vi "ResizeGreyscale.vi"(7 "OpenCV Interpolation Flag":T1, 8 "error in (no error)":errorcluster, 9 "New Image Size":T2, 10 "Greyscale Destination Image":refnum<data-value>, 11 "Greyscale Source Image":refnum<data-value>) -> (0 "error out":errorcluster, 3 "Greyscale Destination Image (duplicate)":refnum<data-value>)   [LabVIEW 2020, in "g_ar_toolkit.image.lvlib"]
uses:
  g_ar_toolkit.image.lvlib
  g_ar_toolkit.common/Image Size (Integer).ctl
  Interpolation Mode.ctl
  eaa3f26c-b51e-4a69-9610-cf2aa5919b39.vi
  <vilib>/Utility/error.llb/Error Cluster From Error Code.vi
  g_ar_toolkit.common/g_ar_toolkit.common.lvlib
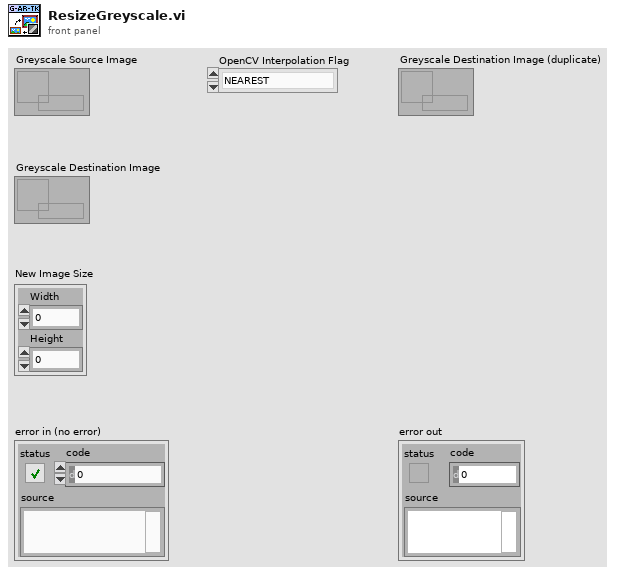
[diagram p1: front panel]
types:
  T1 = typedef "g_ar_toolkit.image.lvlib/Interpolation Mode.ctl" = enum8{"NEAREST", "LINEAR", "CUBIC", "AREA", "LANCZOS", "LINEAR_EXACT", "NEAREST_EXACT", "MAX"}
  T2 = typedef "g_ar_toolkit.common.lvlib/Image Size (Integer).ctl" = cluster{"Width":u16, "Height":u16}
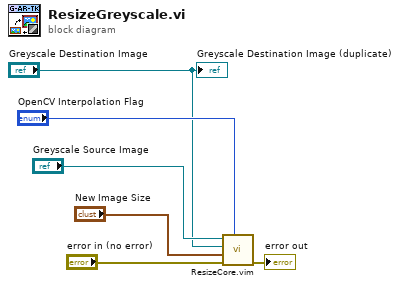
[diagram p0: block diagram]
diagram:
  n1 = call "ResizeCore.vim"("OpenCV Interpolation Flag"="OpenCV Interpolation Flag", "error in (no error)"="error in (no error)", "ImageSize"="New Image Size", "Destination Image"="Greyscale Destination Image", "Source Image"="Greyscale Source Image") -> ("error out"=→"error out":errorcluster)  [unwired: 6 in]
  "Greyscale Destination Image (duplicate)" <- "Greyscale Destination Image"
